vi "Calculate Setpoint.vi"(8 "error in (no error)":errorcluster, 10 "time (sec)":dbl format="%#_13g", 11 "Ramp Setpoint in":refnum<class "Ramp Setpoint.lvclass">) -> (0 "error out":errorcluster, 2 "setpoint":dbl, 3 "Ramp Setpoint out":refnum<class "Ramp Setpoint.lvclass">, 5 "testing?":bool)   [LabVIEW 2020, in "Ramp Setpoint.lvclass"]
uses:
  Ramp Setpoint.lvclass
  C:/Users/jharw/Documents/1 Folder to Rule them All/UMD/Inflation-Apparatus/src/Inflation Test/Parameter Class/IA Test Parameters.lvclass
  Ramp Setpoint.lvclass/Ramp Setpoint.ctl
  IA Test Parameters.lvclass/IA Test Parameters.ctl
  IA Test Parameters.lvclass
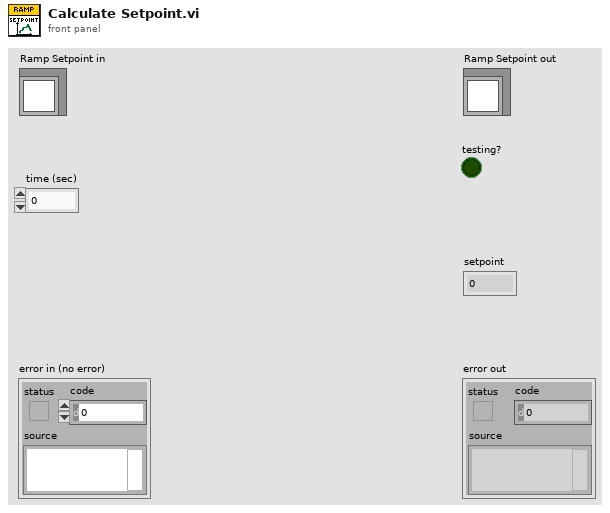
[diagram p1: front panel]
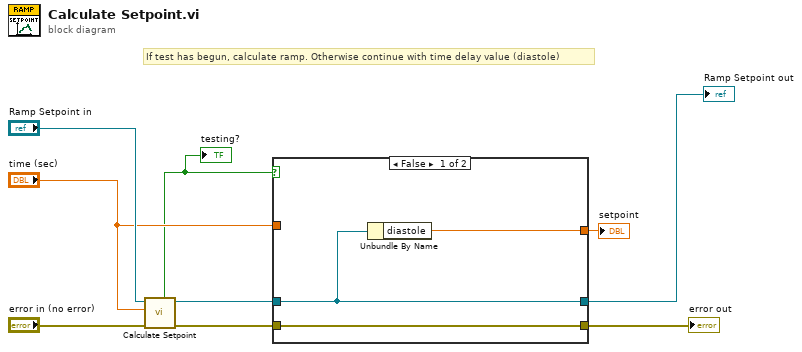
[diagram p0: block diagram]
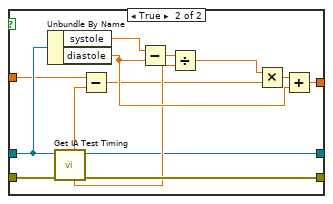
[diagram p2: hidden frame]
diagram:
  # "If test has begun, calculate ramp. Otherwise continue with time delay value (diastole)"
  n1 = call-parent "Calculate Setpoint.vi"("error in (no error)"="error in (no error)", "time (sec)"="time (sec)", "IA Test Parameters in"="Ramp Setpoint in") -> ("error out"=w3:errorcluster, "IA Test Parameters out"=w4:refnum<class "Ramp Setpoint.lvclass">, "testing?"=w6:bool)  [unwired: 5 in, 1 out]
  "testing?" <- w6
  n2 = case shown="False" w6 {
    tunnel: w4 -> [w11 w21]
    tunnel: "time (sec)" -> [_ w17]
    tunnel: [w12 w23] -> w5
    tunnel: w3 -> [w10 w20]
    tunnel: [w10 w19] -> w2
    tunnel: [w11 w13] -> w1
    frame False {
      n3 = Unbundle By Name(w11) -> ("diastole"=w12:dbl)
    }
    frame True {
      n4 = Unbundle By Name(w21) -> ("systole"=w26:dbl, "diastole"=w24:dbl)
      n5 = call "Get IA Test Timing.vi"("error in (no error)"=w20, "IA Test Parameters in"=w21) -> ("error out"=w19:errorcluster, "IA Test Parameters out"=w13:refnum<class "Ramp Setpoint.lvclass">, "test time (sec)"=w18:dbl, "time delay (sec)"=w16:dbl)  [unwired: 4 in, 2 out]
      n6 = Subtract(x=w17, y=w16) -> (x-y=w15:dbl)
      n7 = Subtract(x=w26, y=w24) -> (x-y=w22:dbl)
      n8 = Divide(x=w22, y=w18) -> (x/y=w14:dbl)
      n9 = Multiply(x=w14, y=w15) -> (x*y=w25:dbl)
      n10 = Add(x=w25, y=w24) -> (x+y=w23:dbl)
    }
  }
  "error out" <- w2
  "Ramp Setpoint out" <- w1
  "setpoint" <- w5
